vi "Follow Path.vi"() -> ()   [LabVIEW 2014]
uses:
  navx-mxp/labview/navX-MXP Library/COMMON/TypeDefs/Data TypeDefs/navX YPRH Data.ctl
  navx-mxp/labview/navX-MXP Library/navX-MXP IMU.lvlib
panel:
  out "XY Graph":cluster{dbl[], dbl[]}(graph)
  out "X":dbl
  out "Y":dbl
  out "Reached End":bool
  out "current index value":dbl
  out "Right Motor":dbl(graph)
  out "Left Motor":dbl(graph)
  out "Set Velocity Right":dbl(graph)
  out "Set Velocity Left":dbl(graph)
  out "distance traveled in inches":dbl
  out "distance traveled in feet":dbl
  out "YPRH":T1
  out "PathFileRef":T2
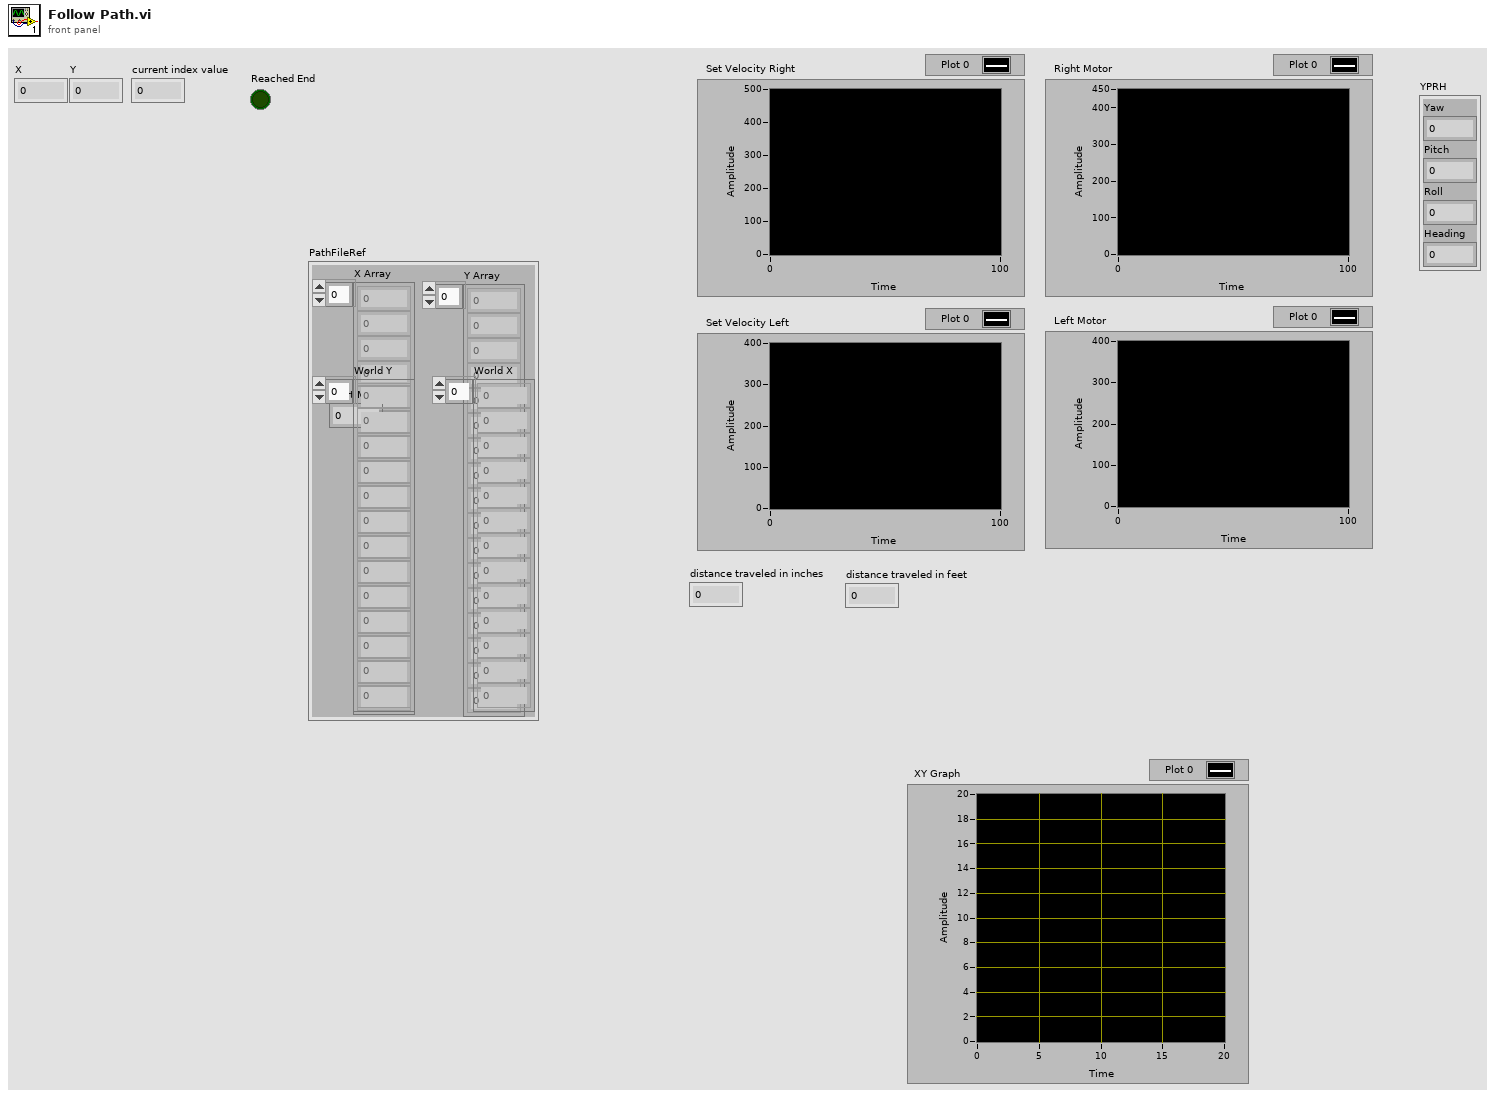
[diagram p1: front panel]
types:
  T1 = typedef "navX-MXP IMU.lvlib/navX YPRH Data.ctl" = cluster{"Yaw":dbl, "Pitch":dbl, "Roll":dbl, "Heading":dbl}
  T2 = cluster{"X Array":dbl[], "Y Array":dbl[], "Start Mill":i32, "World X":dbl[], "World Y":dbl[]}
  T3 = typedef "WPI_MotorControlDeviceRef.ctl" = cluster{"DeviceStatus":errorcluster, "Type":T4, "PWM":cluster{"Controller":T5, "PWM Channel":T6, "DeadBand":T7}, "CAN":cluster{"Device Number":u8, "Control Mode":T8, "Semaphore":T9, "Max Vout":dbl, "TalonSRX Control Mode":T10}, "Invert":bool, "TransformRef":T11, "InvTransformRef":T11}
  T4 = typedef "WPI_MotorControlType.ctl" = enum16{"PWM", "CAN", "CANTalonSRX"}
  T5 = typedef "FPGA_TypedefDigitalModule.ctl" = enum16{"Controller 1"}
  T6 = typedef "FPGA_DIOPWMChannel.ctl" = enum8{"PWM 0", "PWM 1", "PWM 2", "PWM 3", "PWM 4", "PWM 5", "PWM 6", "PWM 7", "PWM 8", "PWM 9", "PWM MXP 0", "PWM MXP 1", "PWM MXP 2", "PWM MXP 3", "PWM MXP 4", "PWM MXP 5", "PWM MXP 6", "PWM MXP 7", "PWM MXP 8", "PWM MXP 9", "Invalid"}
  T7 = typedef "WPI_PWMDeadband.ctl" = cluster{"Name":string, "maxPositivePwm":i32, "minPositivePwm":i32, "centerPwm":i32, "maxNegativePwm":i32, "minNegativePwm":i32, "angularRange":u16}
  T8 = typedef "WPI_CANJaguar_ControlMode.ctl" = enum8{"Percent VBus", "Current", "Speed", "Position", "Voltage"}
  T9 = typedef "Semaphore RefNum" = refnum<k1>
  T10 = typedef "WPI_CANTalonSRX_APIControlMode.ctl" = enum8{"Percent VBus", "Speed", "Position", "Slave", "Unchanged / Invalid"}
  T11 = typedef "WPI_PWMTransform_ConPane.ctl" = refnum<vi>
  T12 = typedef "WPI_CANTalonSRX_GlobalStatus.ctl" = cluster{"Applied Throttle":dbl, "Module Enabled":bool, "CAN Error":errorcluster, "Closed Loop Error":dbl, "Forward Limit Switch Closed":bool, "Reverse Limit Switch Closed":bool, "Sensor Position":dbl, "Sensor Velocity":dbl, "Current":dbl, "Sticky Fault - Over Temp":bool, "Sticky Fault - Under Voltage":bool, "Sticky Fault - Forward Limit":bool, "Sticky Fault - Reverse Limit":bool, "Sticky Fault - Forward Soft Limit":bool, "Sticky Fault - Reverse Soft Limit":bool, "Brake is Enabled":bool, "Encoder Position":dbl, "Encoder Velocity":dbl, "Encoder Index Count":dbl, "Encoder A Pin State":bool, "Encoder B Pin State":bool, "Encoder Index Pin State":bool, "Analog In":dbl, "Analog In Velocity":dbl, "Temperature (C)":dbl, "Battery Voltage":dbl}
  T13 = cluster{"X Array":dbl[], "Y Array":dbl[], "Start Mill":i32, "World X 2":dbl[], "World Y 2":dbl[]}
  T14 = typedef "navX-MXP IMU.lvlib/navX Device TypeDef.ctl" = cluster{"navX Interface Protocol":T15, "navX Interface Protocol TypeDefs":cluster{"SPIDevRef":T16, "I2CDevRef":T18}, "navX System Information":cluster{"Board Information":T20, "Status":T23, "Offsets":T27, "LastSampleTimestamp":dbl, "LastSampleValid":bool}, "navX Common Information":cluster{"Update Rate (4Hz-60Hz)":T28, "refnum name":string, "error":errorcluster, "LastSampleFPGATimestamp":dbl}}
  T15 = typedef "navX-MXP IMU.lvlib/navX Interface Protocol.ctl" = enum16{"SPI", "I2C", "SERIAL"}
  T16 = typedef "WPI_SPIDevRef.ctl" = cluster{"DevStatus":errorcluster, "Handle":i32, "Controller":T5, "SPI Bus":T17}
  T17 = typedef "spi_bus.ctl" = enum16{"SPI On-Board, CS0", "SPI On-Board, CS1", "SPI On-Board, CS2", "SPI On-Board, CS3", "SPI MXP", "Invalid"}
  T18 = typedef "WPI_I2CDevRef.ctl" = cluster{"DevStatus":errorcluster, "Controller":T5, "Device Address":u8, "Handle":i32, "I2C Bus":T19}
  T19 = typedef "i2c_bus.ctl" = enum16{"I2C On-Board", "I2C MXP", "Invalid"}
  T20 = typedef "navX-MXP IMU.lvlib/navX Board Information.ctl" = cluster{"WhoAmI (50 | 0x32)":u8, "Board Revision":u8, "Firmware Major Version":u8, "Firmware Minor Version":u8, "NAVX_BOARD_CAPABILITY":T21, "NAVX_BOARD_YAW_AXIS":T22}
  T21 = typedef "navX-MXP IMU.lvlib/navX NAVX_BOARD_CAPABILITY.ctl" = cluster{"OMNIMOUNT":bool, "YAW_RESET":bool, "VEL_AND_DISP":bool}
  T22 = typedef "navX-MXP IMU.lvlib/navX NAVX_BOARD_YAW_AXIS.ctl" = cluster{"BOARD_YAW_AXIS_UP":bool, "BOARD_YAW_AXIS":u8}
  T23 = typedef "navX-MXP IMU.lvlib/navX Status Data.ctl" = cluster{"Update Rate Hz":u8, "Accelerometer Full-Scale Range":u8, "Gyro Full-Scale Range":u16, "NAVX_OP_STATUS":T24, "NAVX_CAL_STATUS":T25, "NAVX_SELFTEST_STATUS":u8, "NAVX_SENSOR_STATUS":T26}
  T24 = typedef "navX-MXP IMU.lvlib/navX NAVX_OP_STATUS.ctl" = u8
  T25 = typedef "navX-MXP IMU.lvlib/navX NAVX_CAL_STATUS.ctl" = u8
  T26 = typedef "navX-MXP IMU.lvlib/navX NAVX_SENSOR_STATUS.ctl" = cluster{"MOVING":bool, "YAW_STABLE":bool, "MAG_DISTURBANCE":bool, "ALTITUDE_VALID":bool, "SEALEVEL_PRESS_SET":bool, "FUSED_HEADING_VALID":bool}
  T27 = typedef "navX-MXP IMU.lvlib/navX Offsets Data.ctl" = cluster{"Yaw":dbl, "Quat W":dbl, "Quat X":dbl, "Quat Y":dbl, "Quat Z":dbl}
  T28 = typedef "navX-MXP IMU.lvlib/navX Update Rate.ctl" = u8
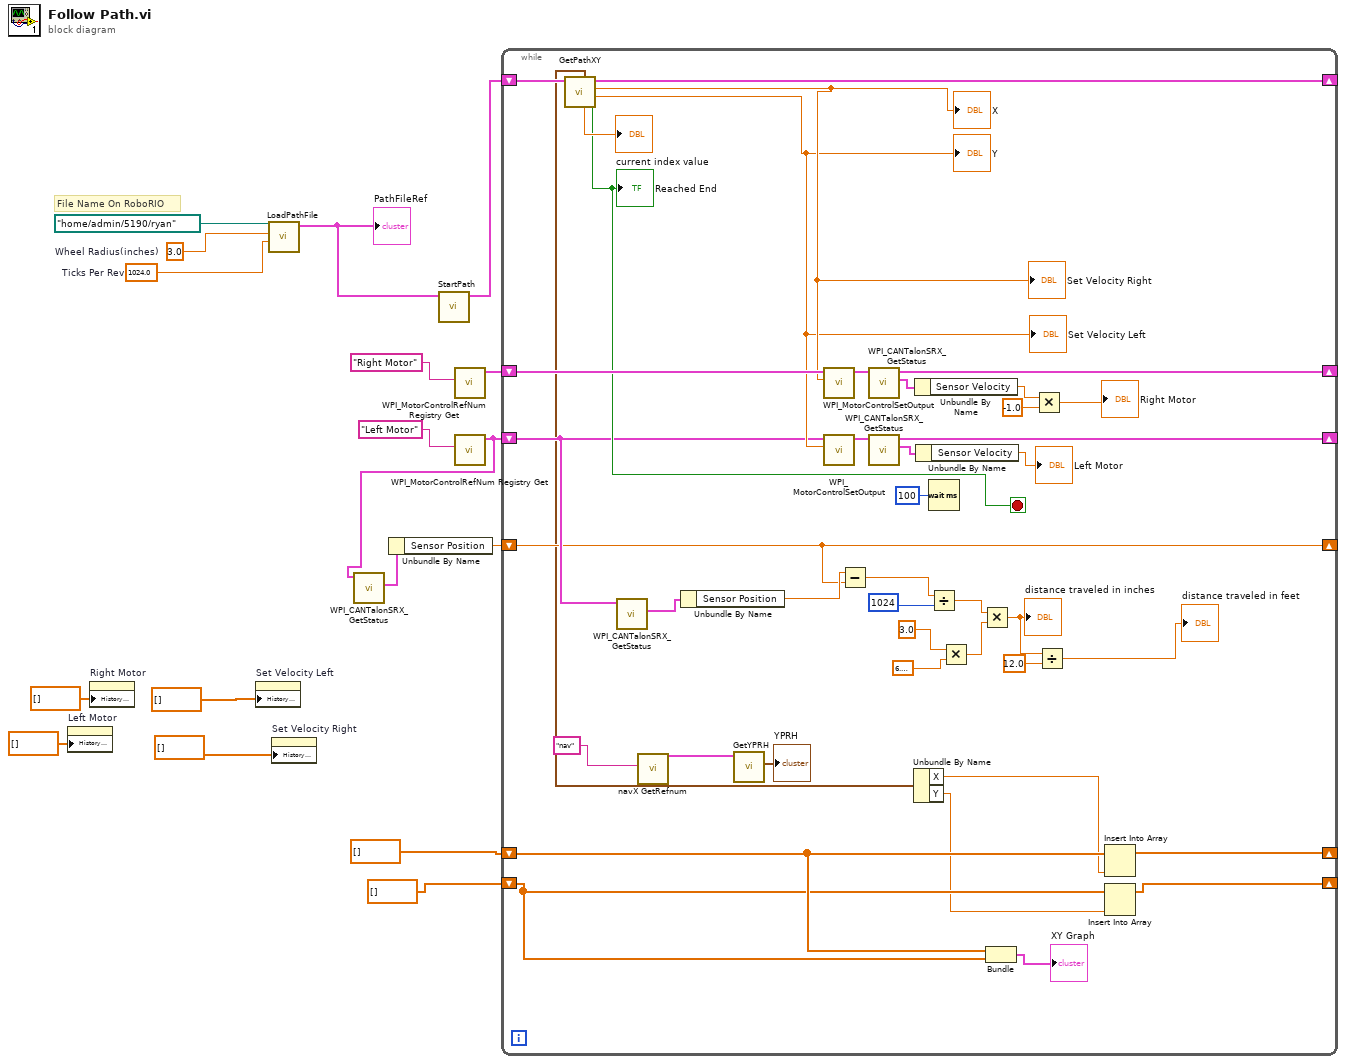
[diagram p0: block diagram]
diagram:
  w15 = 1024.0  # Ticks Per Rev
  w16 = 3.0  # Wheel Radius(inches)
  # "File Name On RoboRIO"
  n1 = property on="Left Motor" class="WFChart (strict)"("History Data"=dbl[] []) -> ()  [unwired: 2 in, 2 out]
  n2 = property on="Right Motor" class="WFChart (strict)"("History Data"=dbl[] []) -> ()  [unwired: 2 in, 2 out]
  n3 = property on="Set Velocity Left" class="WFChart (strict)"("History Data"=dbl[] []) -> ()  [unwired: 2 in, 2 out]
  n4 = call "LoadPathFile.vi"("Ticks Per Rev"=w15, "Wheel Radius(inches)"=w16, "file path (use dialog)"=path "/home/admin/5190/ryan") -> ("PathFileRef"=w14:T2)  [unwired: 8 in]
  "PathFileRef" <- w14
  n5 = property on="Set Velocity Right" class="WFChart (strict)"("History Data"=dbl[] []) -> ()  [unwired: 2 in, 2 out]
  n6 = call "StartPath.vi"("PathFileRef In"=w14) -> ("PathFileRef Out"=w13:T2)  [unwired: 10 in]
  n7 = call <vilib>:"WPI_MotorControlRefNum Registry Get.vi"("refnum name"="Right Motor") -> ("MotorControlDevRef"=w4:T3)  [unwired: 9 in, 1 out]
  n8 = call <vilib>:"WPI_MotorControlRefNum Registry Get.vi"("refnum name"="Left Motor") -> ("MotorControlDevRef"=w3:T3)  [unwired: 9 in, 1 out]
  n9 = call <vilib>:"WPI_CANTalonSRX_GetStatus.vi"("CAN Talon SRX Ref"=w3) -> ("Talon SRX Status"=w6:T12)  [unwired: 8 in, 2 out]
  n10 = Unbundle By Name(w6) -> ("Sensor Position"=w5:dbl)
  n11 = while {
    shift-right: [w58] -> _
    shift-left: w13 -> [w59]
    shift-right: [w53] -> _
    shift-left: w4 -> [w55]
    shift-right: [w51] -> _
    shift-left: w3 -> [w41]
    shift-right: [w38] -> _
    shift-left: w5 -> [w38]
    shift-right: [w21] -> _
    shift-left: dbl[] [] -> [w23]
    shift-right: [w20] -> _
    shift-left: dbl[] [] -> [w19]
    stop <- w45 stop-if-true
    n12 = call "GetPathXY.vi"("PathFileRef In"=w59) -> ("Reached End"=w45:bool, "Y"=w46:dbl, "X"=w47:dbl, "PathFileRef Out"=w58:T13, "current index value"=→"current index value":dbl, "World XY"=w25:cluster{"X":dbl, "Y":dbl})  [unwired: 5 in]
    "X" <- w47
    "Y" <- w46
    "Reached End" <- w45
    "Set Velocity Right" <- w47
    "Set Velocity Left" <- w46
    n13 = call <vilib>:"WPI_CANTalonSRX_GetStatus.vi"("CAN Talon SRX Ref"=w41) -> ("Talon SRX Status"=w40:T12)  [unwired: 8 in, 2 out]
    n14 = call "navX GetRefnum.vi"("refnum name"="nav") -> ("navX Device TypeDef"=w27:T14)  [unwired: 9 in, 1 out]
    n15 = Unbundle By Name(w40) -> ("Sensor Position"=w39:dbl)
    n16 = call "GetYPRH.vi"("navX Device TypeDef"=w27) -> ("YPRH"=→"YPRH":T1)  [unwired: 8 in, 2 out]
    n17 = call <vilib>:"WPI_MotorControlSetOutput.vi"("Output"=w47, "MotorControlDevRef"=w55) -> ("MotorControlDevRef"=w54:T3)  [unwired: 7 in, 2 out]
    n18 = call <vilib>:"WPI_MotorControlSetOutput.vi"("Output"=w46, "MotorControlDevRef"=w41) -> ("MotorControlDevRef"=w52:T3)  [unwired: 7 in, 2 out]
    n19 = Subtract(x=w39, y=w38) -> (x-y=w37:dbl)
    n20 = call <vilib>:"WPI_CANTalonSRX_GetStatus.vi"("CAN Talon SRX Ref"=w54) -> ("Talon SRX Status"=w50:T12, "CAN Talon SRX Ref Out"=w53:T3)  [unwired: 8 in, 1 out]
    n21 = call <vilib>:"WPI_CANTalonSRX_GetStatus.vi"("CAN Talon SRX Ref"=w52) -> ("Talon SRX Status"=w48:T12, "CAN Talon SRX Ref Out"=w51:T3)  [unwired: 8 in, 1 out]
    n22 = Unbundle By Name(w25) -> ("X"=w22:dbl, "Y"=w18:dbl)
    n23 = Unbundle By Name(w50) -> ("Sensor Velocity"=w44:dbl)
    n24 = Unbundle By Name(w48) -> ("Sensor Velocity"=→"Left Motor":dbl)
    n25 = Wait (ms)(milliseconds to wait=u32 100) -> ()  [unwired: 1 out]
    n26 = Divide(x=w37, y=1024) -> (x/y=w33:dbl)
    n27 = Multiply(x=3.0, y=6.283185307179586) -> (x*y=w32:dbl)
    n28 = Multiply(x=w33, y=w32) -> (x*y=w31:dbl)
    "distance traveled in inches" <- w31
    n29 = Bundle(w23, w19) -> (→"XY Graph":cluster{dbl[], dbl[]})  [unwired: 1 in]
    n30 = Multiply(x=w44, y=-1.0) -> (x*y=→"Right Motor":dbl)
    n31 = Divide(x=w31, y=12.0) -> (x/y=→"distance traveled in feet":dbl)
    n32 = Insert Into Array(array=w23, new element=w22) -> (w21:dbl[])  [unwired: 1 in]
    n33 = Insert Into Array(array=w19, new element=w18) -> (w20:dbl[])  [unwired: 1 in]
  }
